vi "RestoreVIWindowTransparency.vi"(7 "VIPath":path, 10 "ErrorIn":errorcluster) -> (2 "ErrorOut":errorcluster)   [LabVIEW 2018]
doc: "Restores the transparency property of the VI specified by <B>VIPath</B> (makes it visible).\n\nUse this after closing another modal window to make a calling VI visible again.\n\nAlso see SetVIWindowTransparency.vi.\n\nCopyright © 2019 Epimedia, Inc. All Rights Reserved.\n\nThe Epimedia Application Library is Copyright © 2009-2017 Epimedia, Inc. \nAll Rights Reserved. Used under license."
panel:
  # "Copyright © 2019 Epimedia, Inc. All Rights Reserved.\n\nThe Epimedia Application Library is Copyright © 2009-2017 Epimedia, Inc. \nAll Rights Reserved. Used under license."
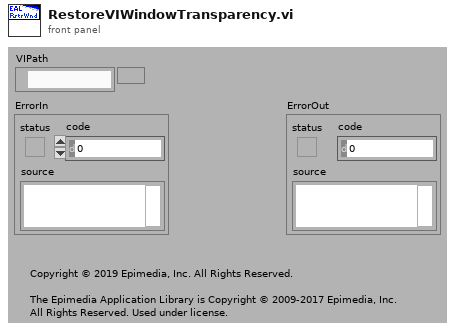
[diagram p1: front panel]
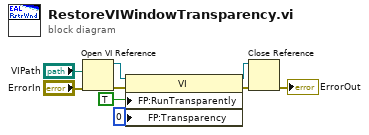
[diagram p0: block diagram]
diagram:
  n1 = Open VI Reference(vi path="VIPath", error in (no error)="ErrorIn") -> (vi reference=w9:refnum<vi>, error out=w8:errorcluster)  [unwired: 4 out]
  n2 = property class="VI"(reference=w9, error in=w8, "FP:RunTransparently"=TRUE ("Front Panel Window:Run VI Transparently"), "FP:Transparency"=u8 0 ("Front Panel Window:Transparency")) -> (reference out=w3:refnum<vi>, error out=w5:errorcluster)
  n3 = Close Reference(reference=w3, error in (no error)=w5) -> (error out=→"ErrorOut":errorcluster)
